vi "dbc-open-frame-tag.vi"(8 "error in (no error)":errorcluster, 11 "dbc in":refnum<class "dbc.lvclass">) -> (0 "error out":errorcluster, 3 "dbc out":refnum<class "dbc.lvclass">)   [LabVIEW 2015, in "dbc.lvclass"]
uses:
  dbc.lvclass
  dbc.lvclass/dbc.ctl
  Read-active-frame-tag.vi
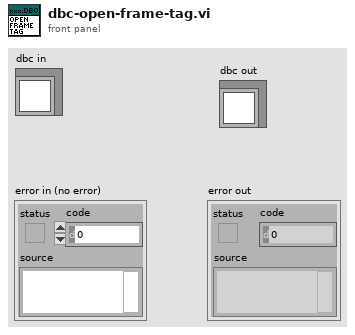
[diagram p1: front panel]
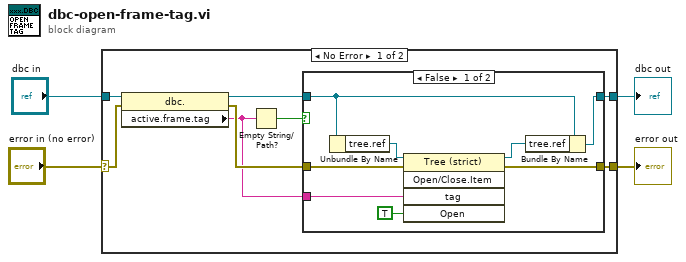
[diagram p0: block diagram]
diagram:
  n1 = case shown="No Error" "error in (no error)" {
    selector: "error in (no error)" -> [w5 w24]
    tunnel: [w10 w24] -> w3
    tunnel: [w9 w23] -> w1
    tunnel: "dbc in" -> [w11 w23]
    frame No Error {
      n2 = property class="dbc."(reference=w11, error in=w5) -> (reference out=w8:refnum<class "dbc.lvclass">, error out=w12:errorcluster, "active.frame.tag"=w6:string)
      n3 = Empty String/Path?(string/path=w6) -> (empty?=w7:bool)
      n4 = case shown="False" w7 {
        tunnel: [w19 w21] -> w10
        tunnel: [w18 w22] -> w9
        tunnel: w12 -> [w16 w21]
        tunnel: w8 -> [w14 w22]
        tunnel: w6 -> [w13 _]
        frame False {
          n5 = Unbundle By Name(w14) -> ("tree.ref"=w15:refnum<vi>)
          n6 = invoke class="Tree (strict)" method="Open/Close.Item"(reference=w15, error in=w16, "tag"=w13, "Open"=TRUE ("Open?")) -> (reference out=w17:refnum<vi>, error out=w19:errorcluster)  [unwired: 1 in, 3 out]
          n7 = Bundle By Name(cluster=w14, "tree.ref"=w17) -> (w18:refnum<class "dbc.lvclass">)
        }
        frame True {
        }
      }
    }
    frame Error {
    }
  }
  "error out" <- w3
  "dbc out" <- w1
